vi "ShowBalloon.vi"(8 "error in (no error)":errorcluster, 10 "Balloon Info":T1, 11 "NotifyIcon in":refnum<class "MGI_TrayIcon.lvclass">) -> (0 "error out":errorcluster, 3 "NotifyIcon out":refnum<class "MGI_TrayIcon.lvclass">)   [LabVIEW 2016, in "MGI_TrayIcon.lvclass"]
doc: "Shows the notification balloon from the tray item.\n\nBalloon Text is required to be a non-empty string. Default timeout is set by the OS, and typically approx 10 sec. For more info see http://msdn.microsoft.com/en-us/library/ms160065.aspx\n\nAuthored by Derek E. Trepanier\nsupport@mooregoodideas.com\nwww.mooregoodideas.com\n\nCopyright (c) 2012, Moore Good Ideas, Inc.\n\nAll rights reserved.\n\nRedistribution and use in source and binary forms, with or without modification, are permitted provided that the following conditions are met:\n\n * Redistributions of source code must retain the above copyright notice, this list of conditions and the following disclaimer.\n * Redistributions in binary form must reproduce the above copyright notice, this list of conditions and the following disclaimer in the documentation and/or other materials provided with the distribution.\n * Neither the name of Moore Good Ideas, Inc. nor the names of its contributors may be used to endorse or promote products derived from this software without specific prior written permission.\n\nTHIS SOFTWARE IS PROVIDED BY THE COPYRIGHT HOLDERS AND CONTRIBUTORS \"AS IS\" AND ANY EXPRESS OR IMPLIED WARRANTIES, INCLUDING, BUT NOT LIMITED TO, THE IMPLIED WARRANTIES OF MERCHANTABILITY AND FITNESS FOR A PARTICULAR PURPOSE ARE DISCLAIMED. IN NO EVENT SHALL THE COPYRIGHT OWNER OR CONTRIBUTORS BE LIABLE FOR ANY DIRECT, INDIRECT, INCIDENTAL, SPECIAL, EXEMPLARY, OR CONSEQUENTIAL DAMAGES (INCLUDING, BUT NOT LIMITED TO, PROCUREMENT OF SUBSTITUTE GOODS OR SERVICES; LOSS OF USE, DATA, OR PROFITS; OR BUSINESS INTERRUPTION) HOWEVER CAUSED AND ON ANY THEORY OF LIABILITY, WHETHER IN CONTRACT, STRICT LIABILITY, OR TORT (INCLUDING NEGLIGENCE OR OTHERWISE) ARISING IN ANY WAY OUT OF THE USE OF THIS SOFTWARE, EVEN IF ADVISED OF THE POSSIBILITY OF SUCH DAMAGE."
uses:
  <userlib>/_MGI/Menu Building/MenuTypes/TrayIcon/MGI_TrayIcon.lvclass
  <userlib>/_MGI/Menu Building/MenuTypes/TrayIcon/BalloonInfo.ctl
  <userlib>/_MGI/Menu Building/MenuTypes/TrayIcon/MGI_TrayIcon.lvclass/MGI_TrayIcon.ctl
  System.Windows.Forms
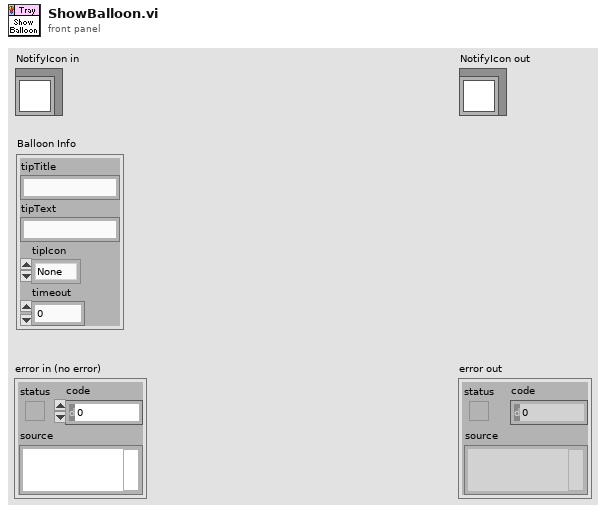
[diagram p1: front panel]
types:
  T1 = typedef "MGI_TrayIcon.lvclass/BalloonInfo.ctl" = cluster{"tipTitle":string, "tipText":string, "tipIcon":enum16{"None", "Info", "Warning", "Error"}, "timeout":i32}
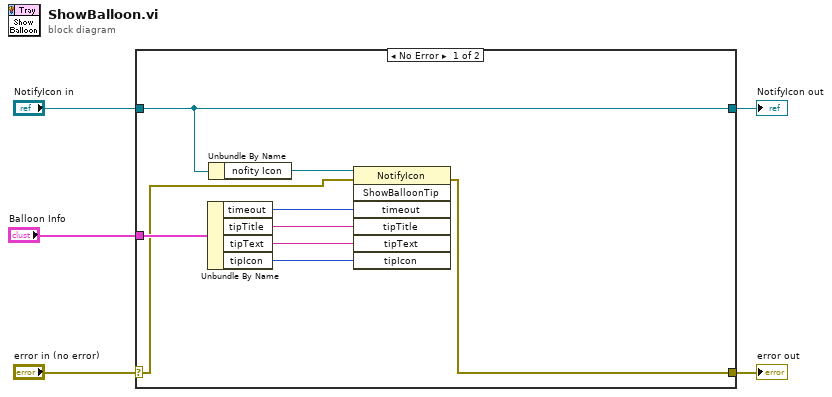
[diagram p0: block diagram]
diagram:
  n1 = case shown="No Error" "error in (no error)" {
    selector: "error in (no error)" -> [w7 w16]
    tunnel: [w6 w16] -> w4
    tunnel: [w14 w15] -> w2
    tunnel: "NotifyIcon in" -> [w14 w15]
    tunnel: "Balloon Info" -> [w12 _]
    frame No Error {
      n2 = Unbundle By Name(w12) -> ("timeout"=w10:i32, "tipTitle"=w9:string, "tipText"=w8:string, "tipIcon"=w11:enum16{"None", "Info", "Warning", "Error"})
      n3 = Unbundle By Name(w14) -> ("nofity Icon"=w13:refnum<k24>)
      n4 = invoke class="NotifyIcon" method="ShowBalloonTip"(reference=w13, error in=w7, "timeout"=w10, "tipTitle"=w9, "tipText"=w8, "tipIcon"=w11) -> (error out=w6:errorcluster)  [unwired: 1 in, 6 out]
    }
    frame Error {
    }
  }
  "error out" <- w4
  "NotifyIcon out" <- w2
